vi "GFVRunForm.vi"(6 "Mode":T1(ring), 7 "表示モード":T2(ring)=enum."Standard", 8 "エラー入力(エラーなし)":errorcluster, 9 "パラメータ(IN)":variant, 11 "VI refnum":refnum<vi>) -> (0 "エラー出力":errorcluster, 1 "パラメータ(OUT)":variant, 2 "REFリスト":refnum<vi>[](array[refnum]), 3 "VI refnum(copy)":refnum<vi>, 4 "タイトルリスト":string[](array[string]), 5 "実行中画面あり?":bool)   [LabVIEW 2014]
panel:
  # "[管理中のウィンドウ一覧]"
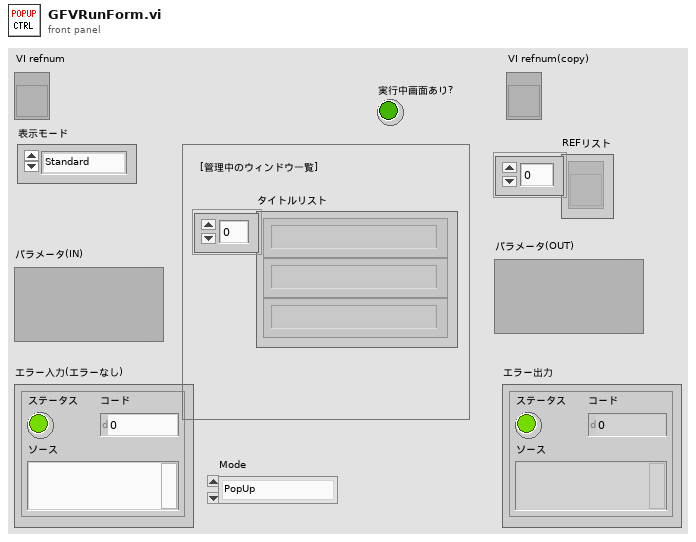
[diagram p1: front panel]
types:
  T1 = enum16{"PopUp", "GetParam", "SetParam", "RunCheck"}
  T2 = enum32{"Invalid", "Standard", "Closed", "Hidden", "Minimized", "Maximized"}
  T3 = enum32{"Bad", "Idle", "Run top level", "Running"}
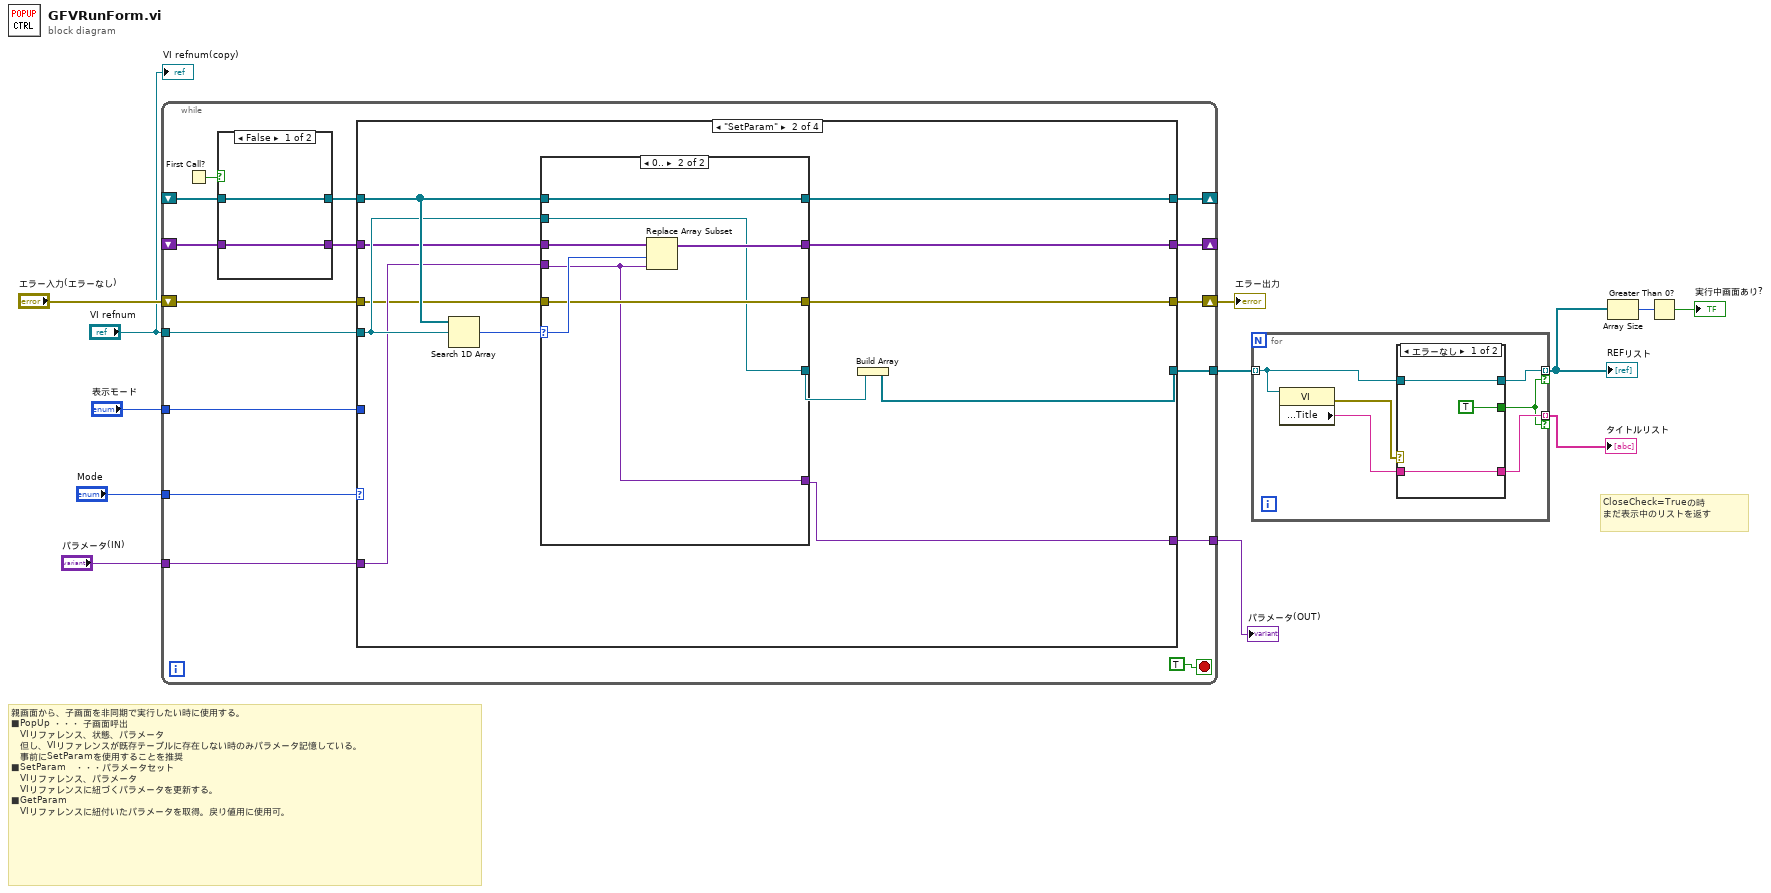
[diagram p0: block diagram]
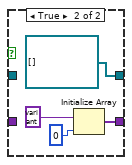
[diagram p3: hidden frame]
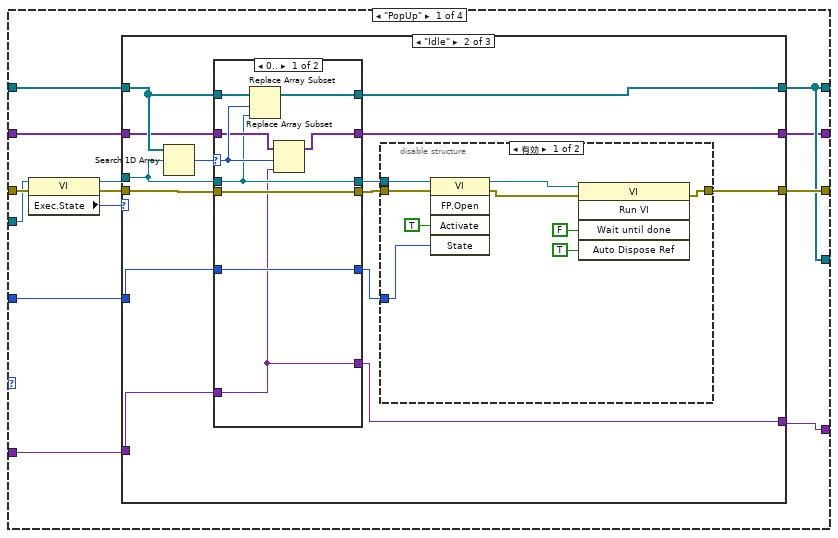
[diagram p4: hidden frame]
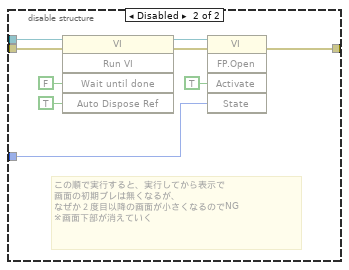
[diagram p6: hidden frame]
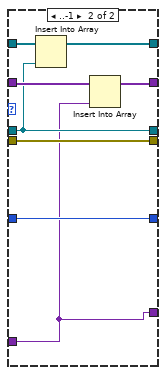
[diagram p7: hidden frame]
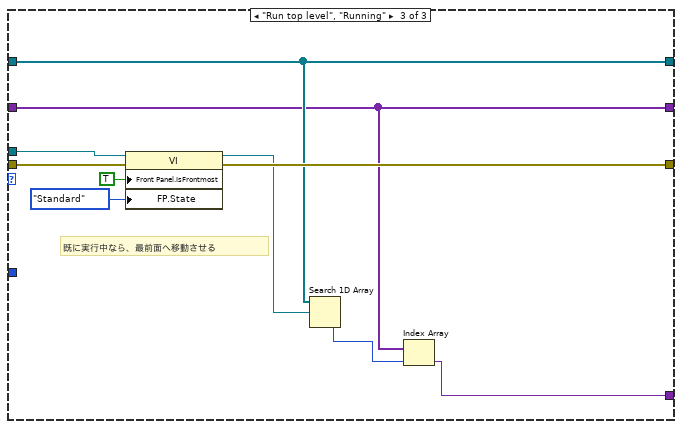
[diagram p8: hidden frame]
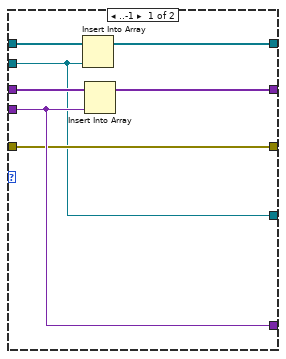
[diagram p9: hidden frame]
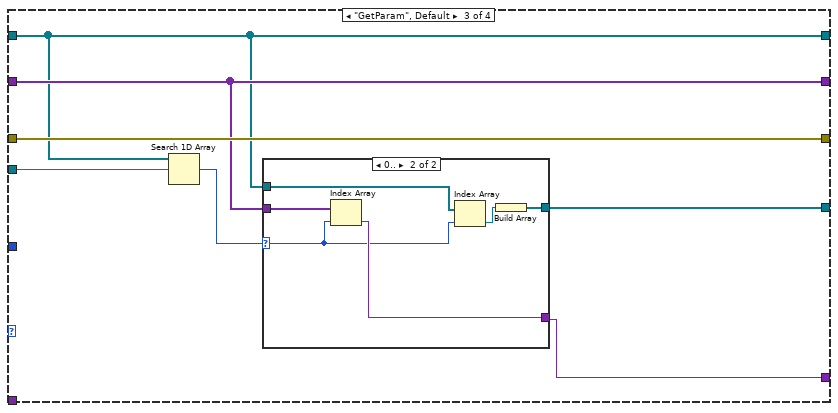
[diagram p10: hidden frame]
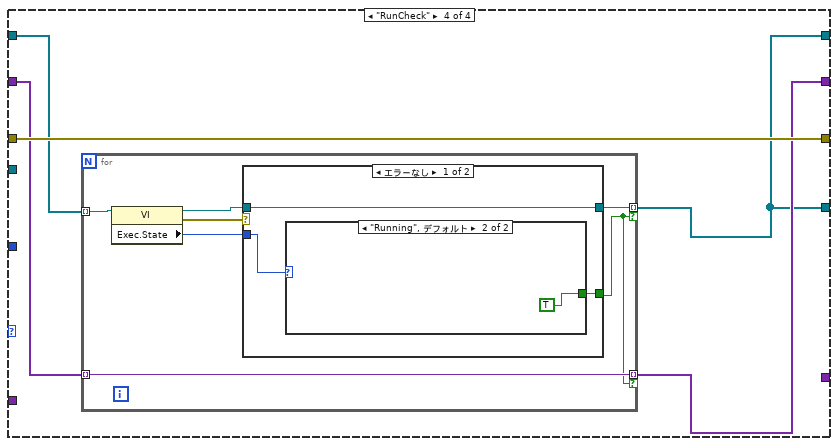
[diagram p12: hidden frame]
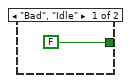
[diagram p13: hidden frame]
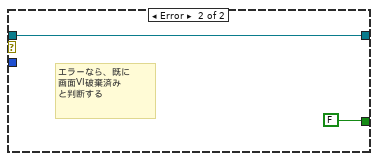
[diagram p14: hidden frame]
diagram:
  # "親画面から、子画面を非同期で実行したい時に使用する。\n■PopUp ・・・ 子画面呼出\n　VIリファレンス、状態、パラメータ\n　但し、VIリファレンスが既存テーブルに存在しない時のみパラメータ記憶している。\n　事前にSetParamを使用することを推奨\n■SetParam　・・・パラメータセット\n　VIリファレンス、パラメータ\n　VIリファレンスに紐づくパラメータを更新する。\n■GetParam \n　VIリファレンスに紐付いたパラメータを取得。戻り値用に使用可。"
  # "CloseCheck=Trueの時\nまだ表示中のリストを返す"
  n1 = while {
    tunnel: "VI refnum" -> [w27]
    tunnel: "表示モード" -> [w25]
    shift-right: [w28] -> w12
    shift-left: "エラー入力(エラーなし)" -> [w26]
    tunnel: "Mode" -> [w23]
    shift-right: [w22] -> _
    shift-left: _ -> [w20]
    tunnel: [w18] -> w8
    tunnel: "パラメータ(IN)" -> [w17]
    shift-right: [w16] -> _
    shift-left: _ -> [w14]
    tunnel: [w13] -> w2
    stop <- TRUE stop-if-true
    n2 = First Call?() -> (First Call?: T/F=w21:bool)
    n3 = case shown="FALSE" w21 {
      tunnel: w20 -> [w30 _]
      tunnel: [w30 refnum<vi>[] []] -> w19
      tunnel: [w29 w33] -> w15
      tunnel: w14 -> [w29 _]
      frame False {
      }
      frame True {
        n4 = Initialize Array(variant ("引数"), 0 ("次元サイズ")) -> (w33:variant[])
      }
    }
    n5 = case shown="\"SetParam\"" w23 {
      tunnel: [w47 w114 w142 w153] -> w28
      tunnel: w27 -> [w35 w119 w141 _]
      tunnel: w26 -> [w46 w113 w142 w153]
      tunnel: w25 -> [w43 _ _ _]
      tunnel: [w41 w116 w137 w149] -> w22
      tunnel: w19 -> [w42 w120 w137 w150]
      tunnel: [w41 w110 w136 w149] -> w18
      tunnel: w17 -> [w38 w117 _ _]
      tunnel: [w40 w115 w138 w151] -> w16
      tunnel: w15 -> [w39 w118 w138 w152]
      tunnel: [w36 w112 w139 _] -> w13
      frame "PopUp" {
        n6 = property class="VI"(reference=w35, error in=w46) -> (reference out=w37:refnum<vi>, error out=w44:errorcluster, "Exec.State"=w45:T3)
        n7 = case shown="\"Idle\"" w45 {
          tunnel: [w50 w54 w106] -> w47
          tunnel: w37 -> [_ w58 w109]
          tunnel: w44 -> [w50 w57 w107]
          tunnel: w43 -> [_ w53 _]
          tunnel: [w49 w64 w105] -> w41
          tunnel: w42 -> [w49 w63 w105]
          tunnel: [w48 w60 w103] -> w40
          tunnel: w39 -> [w48 w61 w103]
          tunnel: w38 -> [_ w59 _]
          tunnel: [_ w51 w101] -> w36
          frame "Bad", Default {
          }
          frame "Idle" {
            n8 = Search 1D Array(1D array=w63, element=w58) -> (index of element=w62:i32)  [unwired: 1 in]
            n9 = case shown="0.." w62 {
              selector: w62 -> [w89 _]
              tunnel: [w90 w99] -> w64
              tunnel: w63 -> [w91 w98]
              tunnel: w58 -> [w86 w95]
              tunnel: w61 -> [w88 w97]
              tunnel: [w87 w96] -> w60
              tunnel: w59 -> [w83 w92]
              tunnel: [w86 w95] -> w55
              tunnel: w57 -> [w85 w94]
              tunnel: [w85 w94] -> w56
              tunnel: [w84 w93] -> w52
              tunnel: w53 -> [w84 w93]
              tunnel: [w83 w92] -> w51
              frame 0.. {
                n10 = Replace Array Subset(array=w91, new element=w86, index=w89) -> (w90:refnum<vi>[])
                n11 = Replace Array Subset(array=w88, new element=w83, index=w89) -> (w87:variant[])
              }
              frame ..-1 {
                n12 = Insert Into Array(array=w98, new element=w95) -> (w99:refnum<vi>[])  [unwired: 1 in]
                n13 = Insert Into Array(array=w97, new element=w92) -> (w96:variant[])  [unwired: 1 in]
              }
            }
            n14 = disable-structure shown="有効" {
              disable-tunnel: w56 -> [w68 w79]
              disable-tunnel: w55 -> [w69 w78]
              disable-tunnel: [w66 w75] -> w54
              disable-tunnel: w52 -> [w70 w74]
              frame Enabled {
                n15 = invoke class="VI" method="FP.Open"(reference=w69, error in=w68, "Activate"=TRUE ("アクティブ化?"), "State"=w70) -> (reference out=w65:refnum<vi>, error out=w67:errorcluster)  [unwired: 1 in, 3 out]
                n16 = invoke class="VI" method="Run VI"(reference=w65, error in=w67, "Wait until done"=FALSE ("終了まで待機"), "Auto Dispose Ref"=TRUE ("リファレンスを自動破棄")) -> (error out=w66:errorcluster)  [unwired: 1 in, 4 out]
              }
              frame Disabled {
                # "この順で実行すると、実行してから表示で\n画面の初期ブレは無くなるが、\nなぜか２度目以降の画面が小さくなるのでNG\n※画面下部が消えていく"
                n17 = invoke class="VI" method="Run VI"(reference=w78, error in=w79, "Wait until done"=FALSE ("終了まで待機"), "Auto Dispose Ref"=TRUE ("リファレンスを自動破棄")) -> (reference out=w76:refnum<vi>, error out=w77:errorcluster)  [unwired: 1 in, 3 out]
                n18 = invoke class="VI" method="FP.Open"(reference=w76, error in=w77, "Activate"=TRUE ("アクティブ化?"), "State"=w74) -> (error out=w75:errorcluster)  [unwired: 1 in, 4 out]
              }
            }
          }
          frame "Run top level", "Running" {
            # "既に実行中なら、最前面へ移動させる"
            n19 = property class="VI"(reference=w109, error in=w107, "Front Panel.IsFrontmost"=TRUE ("フロントパネルウィンドウ:最前面"), "FP.State"=T2."Standard" ("フロントパネルウィンドウ:状態")) -> (reference out=w104:refnum<vi>, error out=w106:errorcluster)
            n20 = Search 1D Array(1D array=w105, element=w104) -> (index of element=w102:i32)  [unwired: 1 in]
            n21 = Index Array(array=w103, index=w102) -> (element=w101:variant)
          }
        }
      }
      frame "SetParam" {
        n22 = Search 1D Array(1D array=w120, element=w119) -> (index of element=w121:i32)  [unwired: 1 in]
        n23 = case shown="0.." w121 {
          selector: w121 -> [_ w132]
          tunnel: w120 -> [w128 w135]
          tunnel: w119 -> [w122 w130]
          tunnel: w118 -> [w127 w134]
          tunnel: w117 -> [w124 w129]
          tunnel: [w126 w135] -> w116
          tunnel: [w125 w133] -> w115
          tunnel: [w123 w131] -> w114
          tunnel: w113 -> [w123 w131]
          tunnel: [w124 w129] -> w112
          tunnel: [w122 w130] -> w111
          frame ..-1 {
            n24 = Insert Into Array(array=w128, new element=w122) -> (w126:refnum<vi>[])  [unwired: 1 in]
            n25 = Insert Into Array(array=w127, new element=w124) -> (w125:variant[])  [unwired: 1 in]
          }
          frame 0.. {
            n26 = Replace Array Subset(array=w134, new element=w129, index=w132) -> (w133:variant[])
          }
        }
        n27 = Build Array(w111) -> (w110:refnum<vi>[])
      }
      frame "GetParam", Default {
        n28 = Search 1D Array(1D array=w137, element=w141) -> (index of element=w140:i32)  [unwired: 1 in]
        n29 = case shown="0.." w140 {
          selector: w140 -> [_ w145]
          tunnel: [_ w147] -> w139
          tunnel: w138 -> [_ w148]
          tunnel: w137 -> [_ w146]
          tunnel: [_ w143] -> w136
          frame ..-1 {
          }
          frame 0.. {
            n30 = Index Array(array=w148, index=w145) -> (element=w147:variant)
            n31 = Index Array(array=w146, index=w145) -> (element=w144:refnum<vi>)
            n32 = Build Array(w144) -> (w143:refnum<vi>[])
          }
        }
      }
      frame "RunCheck" {
        n33 = for {
          tunnel: w150 -> [w160] mode=indexing
          tunnel: [w157] -> w149 mode=indexing if=w154
          tunnel: [w155] -> w151 mode=indexing if=w154
          tunnel: w152 -> [w155] mode=indexing
          n34 = property class="VI"(reference=w160) -> (reference out=w156:refnum<vi>, error out=w159:errorcluster, "Exec.State"=w158:T3)  [unwired: 1 in]
          n35 = case shown="エラーなし" w159 {
            tunnel: w158 -> [w163 _]
            tunnel: [w162 FALSE] -> w154
            tunnel: [w161 w166] -> w157
            tunnel: w156 -> [w161 w166]
            frame No Error {
              n36 = case shown="\"Running\", デフォルト" w163 {
                tunnel: [FALSE TRUE] -> w162
                frame "Bad", "Idle" {
                }
                frame "Running", Default {
                }
              }
            }
            frame Error {
              # "エラーなら、既に\n画面VI破棄済み\nと判断する"
            }
          }
        }
      }
    }
  }
  "エラー出力" <- w12
  "パラメータ(OUT)" <- w2
  n37 = for {
    tunnel: [w169] -> w6 mode=indexing if=w168
    tunnel: w8 -> [w170] mode=indexing
    tunnel: [w171] -> w7 mode=indexing if=w168
    n38 = property class="VI"(reference=w170) -> (error out=w173:errorcluster, "Front Panel.Title"=w172:string)  [unwired: 1 in, 1 out]
    n39 = case shown="エラーなし" w173 {
      tunnel: [w176 _] -> w171
      tunnel: w172 -> [w176 _]
      tunnel: [w175 _] -> w169
      tunnel: w170 -> [w175 _]
      tunnel: [TRUE _] -> w168
      frame No Error {
      }
      frame Error {
      }
    }
  }
  "REFリスト" <- w6
  "タイトルリスト" <- w7
  n40 = Array Size(array=w6) -> (size(s)=w5:i32)
  n41 = Greater Than 0?(x=w5) -> (x > 0?=→"実行中画面あり?":bool)
  "VI refnum(copy)" <- "VI refnum"
